vi "DeStateQueue.vi"(8 "error in (no error)":errorcluster, 11 "QueueIn":variant) -> (0 "error out":errorcluster, 1 "State":T1 caption="States", 3 "QueueOut":variant)   [LabVIEW 2013]
uses:
  SysControl/States.ctl
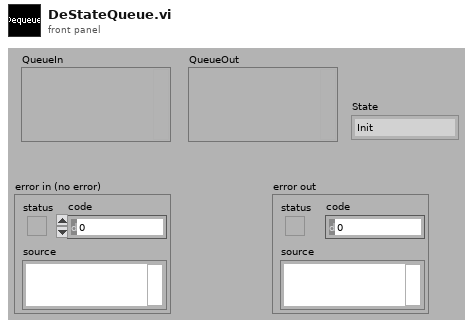
[diagram p1: front panel]
types:
  T1 = typedef "States.ctl" = enum16{"Init", "PreUUT", "Idle", "SetUp", "TestSequence", "PostUUT", "StopTest", "Debug Mode", "Selection Mode", "Loop Mode", "Error", "Wait"}
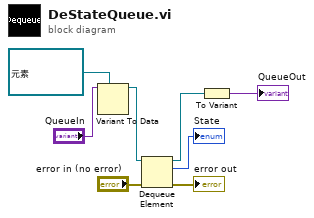
[diagram p0: block diagram]
diagram:
  w4 = refnum<queue> refnum items=["Init", "PreUUT", "Idle", "SetUp", "TestSequence", "PostUUT", "StopTest", "Debug Mode", "Selection Mode", "Loop Mode", "Error", "Wait"] ("队列输出")
  n1 = Variant To Data(type=w4, Variant="QueueIn") -> (data=w5:refnum<queue>)  [unwired: 1 in, 1 out]
  n2 = Dequeue Element(queue=w5, error in (no error)="error in (no error)") -> (queue out=w7:refnum<queue>, element=→"State":T1, error out=→"error out":errorcluster)  [unwired: 2 out]
  n3 = To Variant(anything=w7) -> (Variant=→"QueueOut":variant)
